vi "BigIntIsZero.vi"(1 "a":cluster{"Boolean":bool, "Array":u64[]}) -> (0 "a = 0":bool)   [LabVIEW 2023]
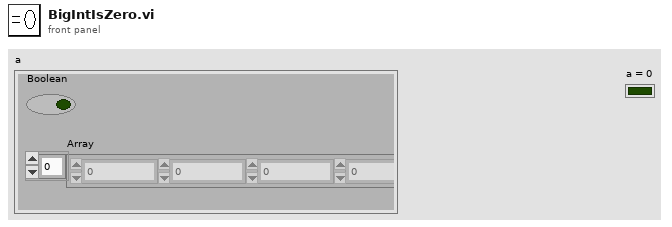
[diagram p1: front panel]
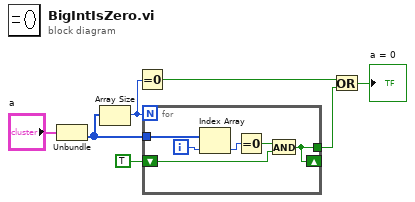
[diagram p0: block diagram]
diagram:
  n1 = Unbundle("a") -> ("Array"=w6:u64[])  [unwired: 1 out]
  n2 = Array Size(array=w6) -> (size(s)=w4:i32)
  n3 = Equal To 0?(x=w4) -> (x = 0?=w3:bool)
  n4 = for {
    N: w4 -> [_]
    tunnel: w6 -> [w12]
    shift-right: [w8] -> _
    shift-left: TRUE -> [w9]
    tunnel: [w8] -> w1
    i -> [w13]
    n5 = Index Array(array=w12, index=w13) -> (element=w10:u64)
    n6 = Equal To 0?(x=w10) -> (x = 0?=w11:bool)
    n7 = And(x=w11, y=w9) -> (x .and. y?=w8:bool)
  }
  n8 = Or(x=w3, y=w1) -> (x .or. y?=→"a = 0":bool)
